vi "Add Defocus and Spherical.vi"(9 "Spherical Comp":dbl, 10 "Defocus Comp":dbl, 11 "Mirror Modes in":T1) -> (3 "Mirror Modes out":T1)   [LabVIEW 2014]
uses:
  DM_Dual_V2/Controls/MirrorModes_DUAL.ctl
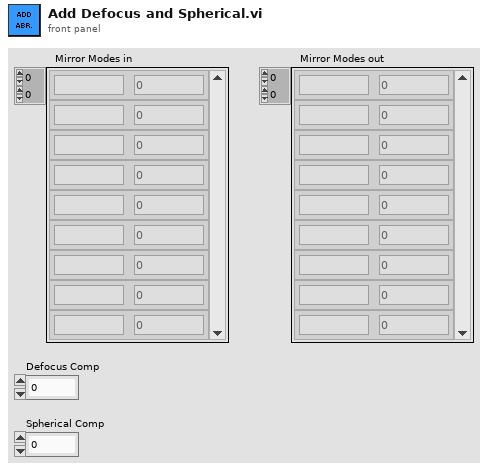
[diagram p1: front panel]
types:
  T1 = typedef "MirrorModes_DUAL.ctl" = cluster{"Mode":string, "Amplitude":dbl}[][]
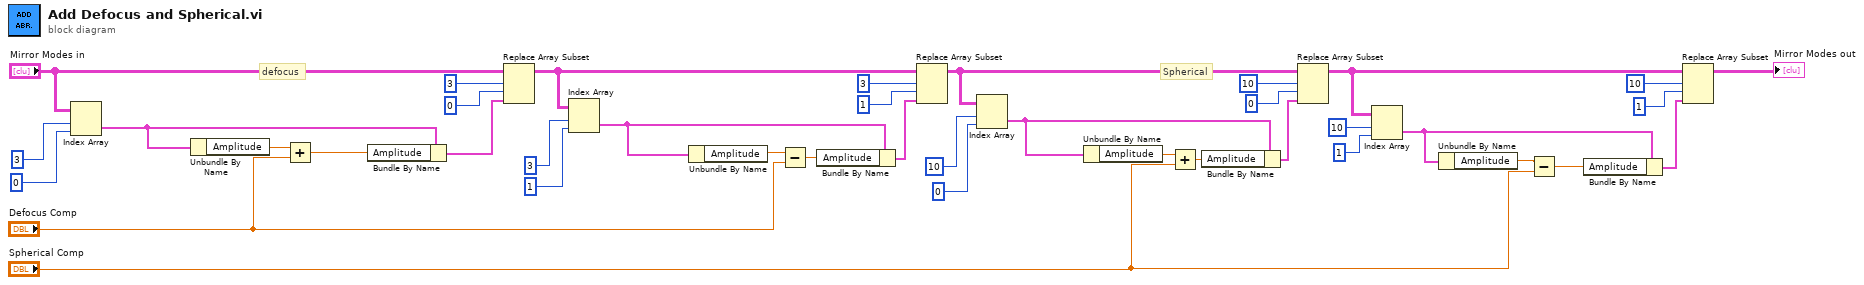
[diagram p0: block diagram]
diagram:
  # "Spherical"
  # "defocus"
  n1 = Index Array(array="Mirror Modes in", index (row)=3 ("disabled index (col)"), index (col)=0 ("disabled index (col)")) -> (element=w7:cluster{"Mode":string, "Amplitude":dbl})
  n2 = Unbundle By Name(w7) -> ("Amplitude"=w20:dbl)
  n3 = Add(x=w20, y="Defocus Comp") -> (x+y=w19:dbl)
  n4 = Bundle By Name(cluster=w7, "Amplitude"=w19) -> (w26:cluster{"Mode":string, "Amplitude":dbl})
  n5 = Replace Array Subset(array="Mirror Modes in", new element=w26, index (row)=3 ("disabled index (row)"), index (col)=0 ("disabled index (col)")) -> (w14:T1)
  n6 = Index Array(array=w14, index (row)=3, index (col)=1 ("disabled index (col)")) -> (element=w6:cluster{"Mode":string, "Amplitude":dbl})
  n7 = Unbundle By Name(w6) -> ("Amplitude"=w15:dbl)
  n8 = Subtract(x=w15, y="Defocus Comp") -> (x-y=w16:dbl)
  n9 = Bundle By Name(cluster=w6, "Amplitude"=w16) -> (w29:cluster{"Mode":string, "Amplitude":dbl})
  n10 = Replace Array Subset(array=w14, new element=w29, index (row)=3, index (col)=1 ("disabled index (col)")) -> (w12:T1)
  n11 = Index Array(array=w12, index (row)=10, index (col)=0 ("disabled index (col)")) -> (element=w5:cluster{"Mode":string, "Amplitude":dbl})
  n12 = Unbundle By Name(w5) -> ("Amplitude"=w9:dbl)
  n13 = Add(x=w9, y="Spherical Comp") -> (x+y=w8:dbl)
  n14 = Bundle By Name(cluster=w5, "Amplitude"=w8) -> (w32:cluster{"Mode":string, "Amplitude":dbl})
  n15 = Replace Array Subset(array=w12, new element=w32, index (row)=10, index (col)=0 ("disabled index (col)")) -> (w35:T1)
  n16 = Index Array(array=w35, index (row)=10, index (col)=1 ("disabled index (col)")) -> (element=w4:cluster{"Mode":string, "Amplitude":dbl})
  n17 = Unbundle By Name(w4) -> ("Amplitude"=w3:dbl)
  n18 = Subtract(x=w3, y="Spherical Comp") -> (x-y=w2:dbl)
  n19 = Bundle By Name(cluster=w4, "Amplitude"=w2) -> (w38:cluster{"Mode":string, "Amplitude":dbl})
  n20 = Replace Array Subset(array=w35, new element=w38, index (row)=10, index (col)=1 ("disabled index (col)")) -> (→"Mirror Modes out":T1)
